vi "GetPhysicalOutputChConfig(AllChannels).vi"(8 "error in (no error)":errorcluster, 11 "Highland T564 DDG in":refnum<class "Highland T564 DDG.lvclass">) -> (0 "error out":errorcluster, 3 "Highland T564 DDG out":refnum<class "Highland T564 DDG.lvclass">)   [LabVIEW 2020, in "Highland T564 DDG.lvclass"]
uses:
  Highland T564 DDG.lvclass
  C:/GEECS/Developers Version/source/Device Drivers/shared/MetaDriver_v1/MetaDriver_v1.lvclass
  Choice84.ctl
  Highland T564 DDG.lvclass/Highland T564 DDG.ctl
  Channel.ctl
  Choice83.ctl
  Choice01.ctl
  T560Session.lvclass
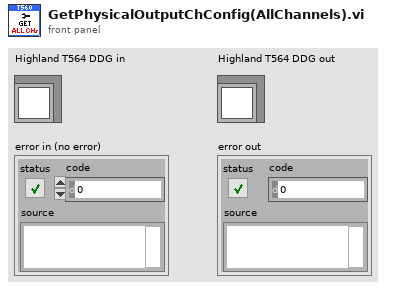
[diagram p1: front panel]
types:
  T1 = typedef "Choice84.ctl" = enum16{"Null", "A", "B", "C", "D", "Trigger"}
  T2 = typedef "Channel.ctl" = cluster{"Polarity":T3, "ChannelOn":enum16{"off", "on"}, "Delay":T4, "Width":T4, "ChannelName":T1}
  T3 = typedef "Choice83.ctl" = enum16{"Direct", "Inverted"}
  T4 = typedef "Choice01.ctl" = cluster{"Value":dbl, "Min":dbl, "Max":dbl, "StepSize":dbl, "Tolerance":dbl, "ValueActual":dbl}
  T5 = typedef "T560Channel.lvclass/ChannelName.ctl" = enum16{"Null", "A", "B", "C", "D", "Trigger"}
  T6 = cluster{"PropertiesAccess:ChannelOn":bool, "PropertiesAccess:Delay":string, "PropertiesAccess:Polarity":enum16{"Direct", "Inverted"}, "PropertiesAccess:Width":string, "ChannelName":T5}
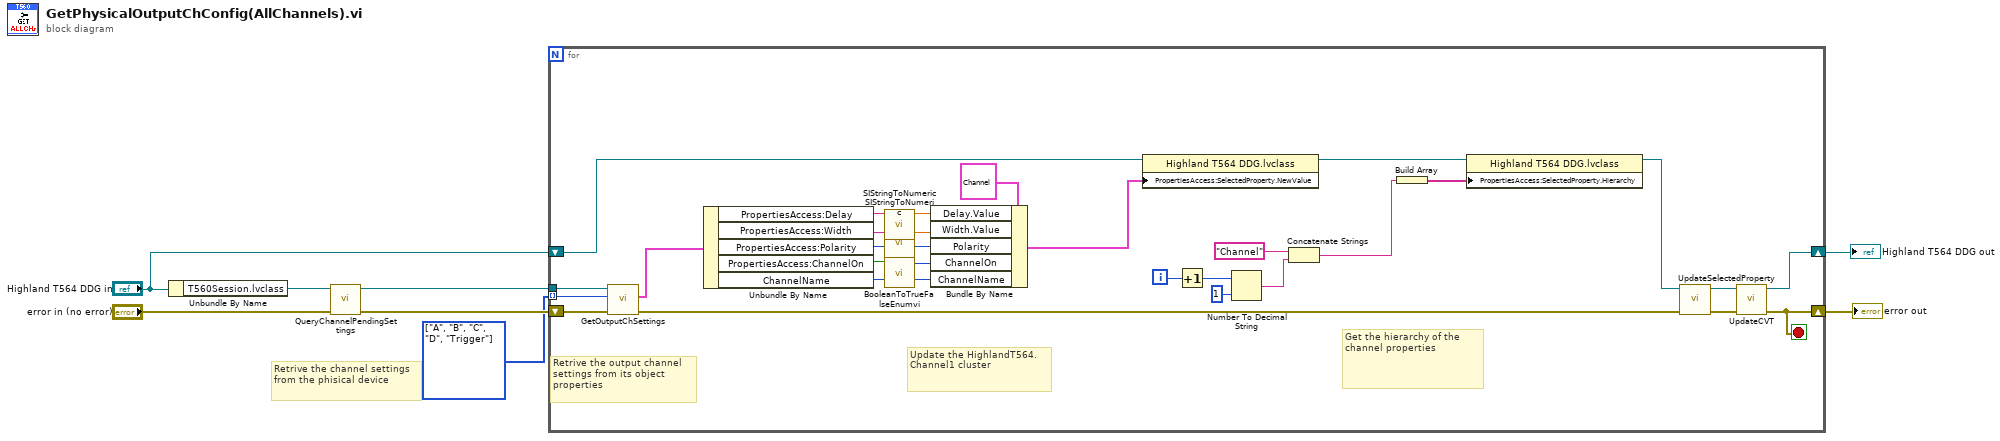
[diagram p0: block diagram]
diagram:
  w5 = T1[] [enum."A", enum."B", enum."C", enum."D", enum."Trigger"] items=["Null", "A", "B", "C", "D", "Trigger"]
  # "Retrive the channel settings from the phisical device"
  n1 = Unbundle By Name("Highland T564 DDG in") -> ("T560Session.lvclass"=w8:refnum<class "T560Session.lvclass">)
  n2 = call-dynamic "QueryChannelPendingSettings.vi"("error in"="error in (no error)", "T560Session in"=w8) -> ("error out"=w6:errorcluster, "T560Session out"=w4:refnum<class "T560Session.lvclass">)  [unwired: 8 in]
  n3 = for {
    tunnel: w4 -> [w32]
    tunnel: w5 -> [w20] mode=indexing
    shift-right: [w9] -> w1
    shift-left: w6 -> [w21]
    shift-right: [w11] -> w2
    shift-left: "Highland T564 DDG in" -> [w19]
    i -> [w18]
    stop <- w9 stop-if-true
    # "Get the hierarchy of the channel properties"
    # "Update the HighlandT564.Channel1 cluster"
    # "Retrive the output channel settings from its object properties"
    n4 = call-dynamic "GetOutputChSettings.vi"("error in (no error)"=w21, "ChannelName"=w20, "T560Session in"=w32) -> ("error out"=w31:errorcluster, "OutputSettings"=w33:T6)  [unwired: 6 in, 1 out]
    n5 = Unbundle By Name(w33) -> ("PropertiesAccess:Delay"=w37:string, "PropertiesAccess:Width"=w35:string, "PropertiesAccess:Polarity"=w29:enum16{"Direct", "Inverted"}, "PropertiesAccess:ChannelOn"=w27:bool, "ChannelName"=w28:T5)
    n6 = call "SIStringToNumeric.vi"("SI number"=w37) -> ("Number"=w36:dbl)  [unwired: 9 in, 1 out]
    n7 = call "SIStringToNumeric.vi"("SI number"=w35) -> ("Number"=w34:dbl)  [unwired: 9 in, 1 out]
    n8 = call "BooleanToTrueFalseEnumvi.vi"("selection"=w27) -> ("On/Off"=w26:enum16{"off", "on"})  [unwired: 10 in]
    n9 = Bundle By Name(cluster=T2 {"Polarity"=enum."Direct", "ChannelOn"=enum."off", "Delay"={"Value"=0.0, "Min"=0.0, "Max"=0.0, "StepSize"=0.0, "Tolerance"=0.0, "ValueActual"=0.0}, "Width"={"Value"=0.0, "Min"=0.0, "Max"=0.0, "StepSize"=0.0, "Tolerance"=0.0, "ValueActual"=0.0}, "ChannelName"=enum."Null"} ("Channel1"), "Delay.Value"=w36, "Width.Value"=w34, "Polarity"=w29, "ChannelOn"=w26, "ChannelName"=w28) -> (w25:T2)
    n10 = property class="Highland T564 DDG.lvclass"(reference=w19, "PropertiesAccess:SelectedProperty.NewValue"=w25) -> (reference out=w24:refnum<class "Highland T564 DDG.lvclass">)  [unwired: 1 in, 1 out]
    n11 = Increment(x=w18) -> (x+1=w17:i32)
    n12 = Number To Decimal String(number=w17, width (-)=i16 1) -> (decimal integer string=w15:string)
    n13 = Concatenate Strings("Channel", w15) -> (w13:string)
    n14 = Build Array(w13) -> (w22:string[])
    n15 = property class="Highland T564 DDG.lvclass"(reference=w24, "PropertiesAccess:SelectedProperty.Hierarchy"=w22) -> (reference out=w23:refnum<class "Highland T564 DDG.lvclass">)  [unwired: 1 in, 1 out]
    n16 = call-dynamic "UpdateSelectedProperty.vi"("error in (no error)"=w31, "Highland T564 DDG in"=w23) -> ("error out"=w10:errorcluster, "Highland T564 DDG out"=w12:refnum<class "Highland T564 DDG.lvclass">)  [unwired: 8 in]
    n17 = call-dynamic "UpdateCVT.vi"("error in (no error)"=w10, "Highland T564 DDG in"=w12) -> ("error out"=w9:errorcluster, "Highland T564 DDG out"=w11:refnum<class "Highland T564 DDG.lvclass">)  [unwired: 8 in]
  }
  "Highland T564 DDG out" <- w2
  "error out" <- w1
